vi "Global Variables.vi"() -> ()   [LabVIEW 2024]
uses:
  RecipeEditor Actor/Setting.ctl
panel:
  out "Torque(Nm) Load":dbl
  out "4503#0Ready":bool
  in  "TestData":string
  out "Torque(Nm)":dbl
  in  "Setting":T1={"TorqueSensor"={"Interface"="", "Read Unit"=enum."Kg.cm", "Encoder"=0, "Torque Filter"=0, "Max Torque"=2.0, "Max Power"=50.0, "Max Speed"=50.0, "Scale Factor CW"=2.0, "Scale Factor CCW"=2.0, "Scale Factor Zero"=2.0}, "DC-1000"={"Interface"=enum."AD-1"}, "ServoMotor"={"Interface"=enum."AD-1"}} {"TorqueSensor"."Scale Factor Zero" format="%#.6f"; "TorqueSensor"."Scale Factor CCW" format="%#.6f"; "TorqueSensor"."Scale Factor CW" format="%#.6f"; "TorqueSensor"."Torque Filter" items=["OFF", "10Hz", "25Hz", "50Hz", "3Hz", "2Hz", "1Hz"]; "TorqueSensor"."Encoder" items=["60-ppr"=60, "600-ppr"=600, "6000-ppr"=6000, "8192-ppr"=8192, "20-ppr"=20, "30-ppr"=30, "1-ppr"=1, "2-ppr"=2, "6-ppr"=6]}
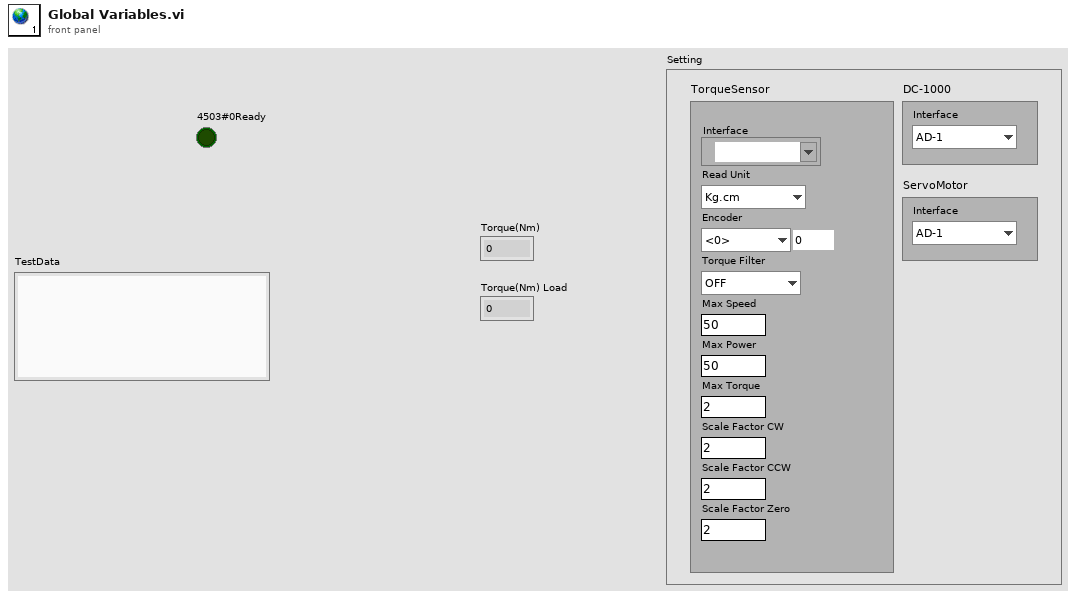
[diagram p1: front panel]
types:
  T1 = typedef "Setting.ctl" = cluster{"TorqueSensor":cluster{"Interface":refnum<visa-resource-name>, "Read Unit":enum16{"oz.in", "oz.ft", "lb.in", "lb.ft", "g.cm", "Kg.cm", "mN.m", "cN.m", "N.m"}, "Encoder":u16, "Torque Filter":u16, "Max Torque":dbl, "Max Power":dbl, "Max Speed":dbl, "Scale Factor CW":dbl, "Scale Factor CCW":dbl, "Scale Factor Zero":dbl}, "DC-1000":cluster{"Interface":enum16{"AD-0", "AD-1"}}, "ServoMotor":cluster{"Interface":enum16{"AD-0", "AD-1"}}}
diagram:
